vi "Actor Core.vi"(8 "error in":errorcluster, 11 "TCPIP Reader in":refnum<class "TCPIP Reader.lvclass">) -> (0 "error out":errorcluster, 3 "Actor out":refnum<class "Actor.lvclass">)   [LabVIEW 2015, in "TCPIP Reader Actor.lvlib" / "TCPIP Reader.lvclass"]
doc: "(<B>Filename</B>: Actor Framework.lvlib:Actor.lvclass:Actor Core.vi)\n\nReceives messages to the actor, reacts to them, and initiates any error handling that may shut the actor down.\n\nDescendant classes may override this VI to append parallel tasks for the actor to complete while it handles messages. Overrides use the Call Parent Method node."
uses:
  TCPIP Reader.lvclass
  <vilib>/ActorFramework/Actor/Actor.lvclass
  TCPIP Reader.lvclass/TCPIP Reader.ctl
  <vilib>/ActorFramework/Actor/Actor.lvclass/Actor.ctl
  <vilib>/ActorFramework/Message Enqueuer/Message Enqueuer.lvclass/Message Enqueuer.ctl
  TCPIP Communications Framework/TCPIP Communications Messages/Close Communications Msg/Close Communications Msg.lvclass/Close Communications Msg.ctl
  <vilib>/ActorFramework/Message Enqueuer/Init from Existing Queue.vi
  <vilib>/ActorFramework/Message Enqueuer/Enqueue.vi
  <vilib>/ActorFramework/Message Priority Queue/Priority Enqueue.vi
  <vilib>/ActorFramework/Message Enqueuer/Message Enqueuer.lvclass
  TCPIP Communications Framework/TCPIP Communications Messages/Close Communications Msg/Close Communications Msg.lvclass
  <vilib>/ActorFramework/Stop Msg/Stop Msg.lvclass
  TCPIP Communications Framework/TCPIP Communications Messages/Packet Msg/Packet Msg.lvclass
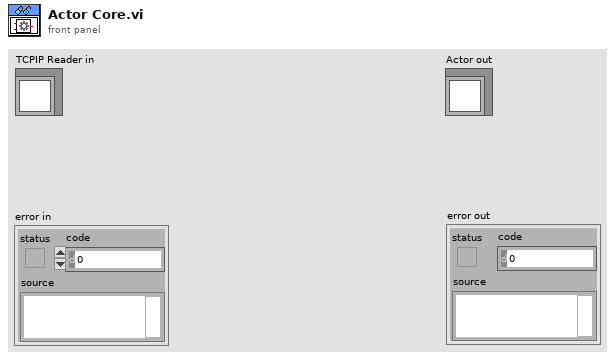
[diagram p1: front panel]
types:
  T1 = enum16{"big-endian, network order", "native, host order", "little-endian"}
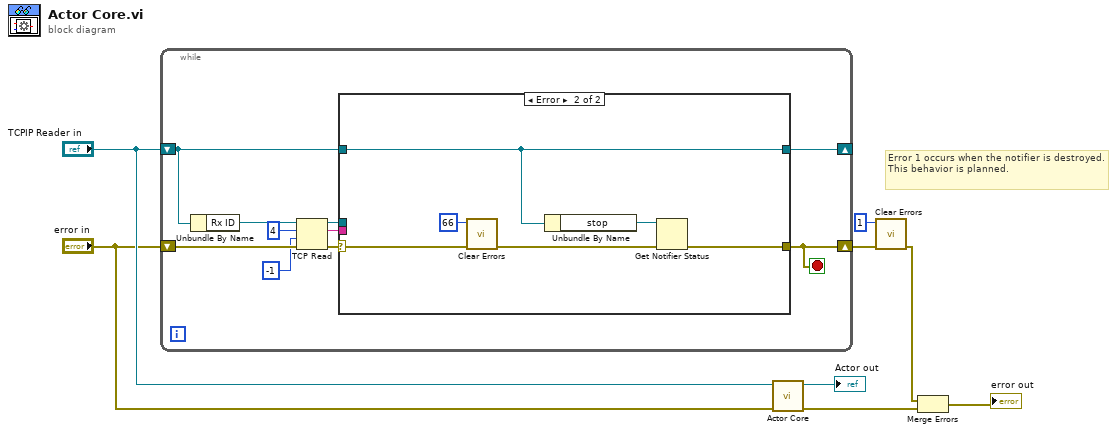
[diagram p0: block diagram]
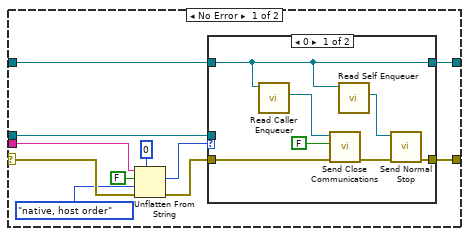
[diagram p2: hidden frame]
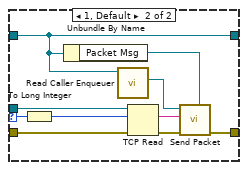
[diagram p3: hidden frame]
diagram:
  # "Error 1 occurs when the notifier is destroyed. This behavior is planned."
  n1 = while {
    shift-right: [w10] -> w4
    shift-left: "error in" -> [w17]
    shift-right: [w9] -> _
    shift-left: "TCPIP Reader in" -> [w18]
    stop <- w10 stop-if-true
    n2 = Unbundle By Name(w18) -> ("Rx ID"=w15:refnum<k5>)
    n3 = TCP Read(connection ID=w15, bytes to read=4, error in (no error)=w17, 9:-1 ("timeout ms (25000)")) -> (connection ID out=w13:refnum<k5>, data out=w12:string, error out=w14:errorcluster)  [unwired: 1 in]
    n4 = case shown="Error" w14 {
      selector: w14 -> [w26 w52]
      tunnel: w13 -> [w25 _]
      tunnel: w12 -> [w27 _]
      tunnel: w18 -> [w23 w50]
      tunnel: [w20 w50] -> w9
      tunnel: [w22 w47] -> w10
      frame No Error {
        n5 = Unflatten From String(type=u32 0 ("bytes to read"), binary string=w27, data includes array or string size? (T)=FALSE, byte order (0:big-endian, network order)=T1."native, host order", error in (no error)=w26) -> (value=w21:u32, error out=w24:errorcluster)  [unwired: 1 out]
        n6 = case shown="0" w21 {
          selector: w21 -> [_ w40]
          tunnel: w25 -> [_ w46]
          tunnel: w24 -> [w35 w45]
          tunnel: w23 -> [w33 w38]
          tunnel: [w30 w41] -> w22
          tunnel: [w33 w38] -> w20
          frame 0 {
            n7 = call <vilib>:"Read Caller Enqueuer.vi"("Actor"=w33) -> ("Caller Enqueuer"=w34:refnum<class "Message Enqueuer.lvclass">)  [unwired: 10 in]
            n8 = call "Send Close Communications.vi"("error in (no error)"=w35, "Final Stop?"=FALSE, "Message Enqueuer"=w34) -> ("error out"=w32:errorcluster)  [unwired: 7 in, 1 out]
            n9 = call <vilib>:"Read Self Enqueuer.vi"("Actor"=w33) -> ("Self Enqueuer"=w31:refnum<class "Message Enqueuer.lvclass">)  [unwired: 10 in]
            n10 = call <vilib>:"Send Normal Stop.vi"("error in (no error)"=w32, "Message Enqueuer"=w31) -> ("error out"=w30:errorcluster)  [unwired: 9 in]
          }
          frame 1, Default {
            n11 = To Long Integer(number=w40) -> (32bit integer=w39:i32)
            n12 = Unbundle By Name(w38) -> ("Packet Msg"=w42:refnum<class "Packet Msg.lvclass">)
            n13 = call <vilib>:"Read Caller Enqueuer.vi"("Actor"=w38) -> ("Caller Enqueuer"=w37:refnum<class "Message Enqueuer.lvclass">)  [unwired: 10 in]
            n14 = TCP Read(connection ID=w46, bytes to read=w39, error in (no error)=w45) -> (data out=w44:string, error out=w43:errorcluster)  [unwired: 2 in, 1 out]
            n15 = call "Send Packet.vi"("Packet Msg"=w42, "error in (no error)"=w43, "Packet"=w44, "Message Enqueuer in"=w37) -> ("error out"=w41:errorcluster)  [unwired: 6 in, 1 out]
          }
        }
      }
      frame Error {
        n16 = call <vilib>:"Clear Errors.vi"("error in (no error)"=w52, "specific error code to clear (0: all)"=66) -> ("error out"=w48:errorcluster)  [unwired: 4 in, 1 out]
        n17 = Unbundle By Name(w50) -> ("stop"=w49:refnum<notifier>)
        n18 = Get Notifier Status(notifier=w49, error in (no error)=w48) -> (error out=w47:errorcluster)  [unwired: 4 out]
      }
    }
  }
  n19 = call-parent "Actor Core.vi"("error in"="error in", "Actor in"="TCPIP Reader in") -> ("error out"=w3:errorcluster, "Actor out"=→"Actor out":refnum<class "Actor.lvclass">)  [unwired: 8 in]
  n20 = call <vilib>:"Clear Errors.vi"("error in (no error)"=w4, "specific error code to clear (0: all)"=1) -> ("error out"=w2:errorcluster)  [unwired: 4 in, 1 out]
  n21 = Merge Errors(w2, w3) -> (→"error out":errorcluster)
